vi "MoveMultiDrives.vi"(0 "Start Counter":dbl[](array[numeric]), 1 "Matched Configurations In":T2[](array[typedef]) {"Static Drive Configuration"."Indexer Mode  (FSA)" items=["Incremental", "Absolute"]; "Static Drive Configuration"."Buffer at Stop (SSH)" items=["Clear buffer", "Save and Continue"]; "Static Drive Configuration"."Buffer at Limit (SSG)" items=["Clear buffer", "Save and Continue"]; "Static Drive Configuration"."RS232 Echo Control (SSA)" items=["Echo ON", "Echo OFF"]; "Static Drive Configuration"."Reference edge of Home (OSH)" items=["CW", "CCW"]; "Static Drive Configuration"."Encoder Z for Home (OSD)" items=["Don't use", "Enable"]; "Static Drive Configuration"."Home Switch Sense (OSC)" items=["Normally Open", "Normally Closed"]; "Static Drive Configuration"."Home Position (OSB)" items=["Anywhere in Switch", "Edge of Switch"]; "Static Drive Configuration"."Limit Switch Sense (OSA)" items=["Normally Closed", "Normally Open"]; "Static Drive Configuration"."Limit Disable (LD)" items=["Both Enabled", "CW Disabled", "CCW Disabled", "Both Disabled"]; "Static Drive Configuration"."Stall Detect (FSH)" items=["Disable", "Enable"]; "Static Drive Configuration"."OP2 in Deadband (FSG)" items=["Don't Use", "ACTIVATE"]; "Static Drive Configuration"."Stop on Trigger 3 (FSF)" items=["Ignore", "STOP!"]; "Static Drive Configuration"."Activate OP1 on stall (FSE)" items=["Do not Activate", "ACTIVATE!"]; "Static Drive Configuration"."Stop on Stall (FSD)" items=["Continue", "STOP"]; "Static Drive Configuration"."Position Maintenance (FSC)" items=["Disabled", "Enabled"]; "Static Drive Configuration"."Step Mode  (FSB)" items=["Motor", "Encoder"]; "Static Drive Configuration"."Encoder Resolution (ER)" min=1 max=50000; "Static Drive Configuration"."Dead Band Window (DW)" min=0 max=999999999; "Static Drive Configuration"."Dead Band (DB)" min=0 max=999999999; "Static Drive Configuration"."Correction Gain % (CG)" items=["n/a", "12.5", "25", "37.5", "50", "62.5", "75", "87.5", "100"]; "Channel Properties"."Current Pos" format="%.2f"; "Channel Properties"."Backlash/Eng units" format="%.2f"; "Channel Properties"."Pulses/rev" format="%.2f"; "Channel Properties"."Pos Tolerance" format="%.2f"; "Channel Properties"."Pulses/unit" format="%.2f"; "Channel Properties"."Acc. Min" format="%.2f"; "Channel Properties"."Acc. Max" format="%.2f"; "Channel Properties"."Vel. Min" format="%.2f"; "Channel Properties"."Vel. Max" format="%.2f"; "Channel Properties"."Acc. Default" format="%.2f"; "Channel Properties"."Vel. Default" format="%.2f"}, 2 "GoTo Array (pulse position some channels)":T5[](array[typedef]) {"Acceleration" format="%.2f"; "Velocity" format="%.2f"; "Go To Position" step=100000.0}, 3 "Final move":bool, 4 "Predicted Move Time":dbl format="%.2f") -> (5 "Error string":string, 6 "Stop Pressed?":bool, 7 "Matched Configurations Out":T2[](array[typedef]) {"Static Drive Configuration"."Indexer Mode  (FSA)" items=["Incremental", "Absolute"]; "Static Drive Configuration"."Buffer at Stop (SSH)" items=["Clear buffer", "Save and Continue"]; "Static Drive Configuration"."Buffer at Limit (SSG)" items=["Clear buffer", "Save and Continue"]; "Static Drive Configuration"."RS232 Echo Control (SSA)" items=["Echo ON", "Echo OFF"]; "Static Drive Configuration"."Reference edge of Home (OSH)" items=["CW", "CCW"]; "Static Drive Configuration"."Encoder Z for Home (OSD)" items=["Don't use", "Enable"]; "Static Drive Configuration"."Home Switch Sense (OSC)" items=["Normally Open", "Normally Closed"]; "Static Drive Configuration"."Home Position (OSB)" items=["Anywhere in Switch", "Edge of Switch"]; "Static Drive Configuration"."Limit Switch Sense (OSA)" items=["Normally Closed", "Normally Open"]; "Static Drive Configuration"."Limit Disable (LD)" items=["Both Enabled", "CW Disabled", "CCW Disabled", "Both Disabled"]; "Static Drive Configuration"."Stall Detect (FSH)" items=["Disable", "Enable"]; "Static Drive Configuration"."OP2 in Deadband (FSG)" items=["Don't Use", "ACTIVATE"]; "Static Drive Configuration"."Stop on Trigger 3 (FSF)" items=["Ignore", "STOP!"]; "Static Drive Configuration"."Activate OP1 on stall (FSE)" items=["Do not Activate", "ACTIVATE!"]; "Static Drive Configuration"."Stop on Stall (FSD)" items=["Continue", "STOP"]; "Static Drive Configuration"."Position Maintenance (FSC)" items=["Disabled", "Enabled"]; "Static Drive Configuration"."Step Mode  (FSB)" items=["Motor", "Encoder"]; "Static Drive Configuration"."Encoder Resolution (ER)" min=1 max=50000; "Static Drive Configuration"."Dead Band Window (DW)" min=0 max=999999999; "Static Drive Configuration"."Dead Band (DB)" min=0 max=999999999; "Static Drive Configuration"."Correction Gain % (CG)" items=["n/a", "12.5", "25", "37.5", "50", "62.5", "75", "87.5", "100"]; "Channel Properties"."Current Pos" format="%.2f"; "Channel Properties"."Backlash/Eng units" format="%.2f"; "Channel Properties"."Pulses/rev" format="%.2f"; "Channel Properties"."Pos Tolerance" format="%.2f"; "Channel Properties"."Pulses/unit" format="%.2f"; "Channel Properties"."Acc. Min" format="%.2f"; "Channel Properties"."Acc. Max" format="%.2f"; "Channel Properties"."Vel. Min" format="%.2f"; "Channel Properties"."Vel. Max" format="%.2f"; "Channel Properties"."Acc. Default" format="%.2f"; "Channel Properties"."Vel. Default" format="%.2f"})   [LabVIEW 2010]
uses:
  ~subVIs/DriveClusterLower.ctl
  ~subVIs/AxisConfigCluster.ctl
  ~subVIs/DriveProperties.ctl
  ~subVIs/DriveStaticConfig.ctl
  ~subVIs/DriveStatus.ctl
  ~subVIs/GenericDriveCommand.ctl
  ~subVIs/DriveConfigGlobal.vi
panel:
  out "Server copy Location":path
  out "Log File":path
  out "Move Terminated on Timeout":bool
  in  "Axis info cluster":T1
  out "Start Time":dbl format="%.2f"
  out "Running":bool
  out "Bar2":dbl(slide)=2.0 scale=0.0..-50.0
  out "Bar1":dbl(slide)=2.0 scale=34109.0..-5753.438776987422
  out "Bar0":dbl(slide)=2.0 scale=204595.2..204800.0
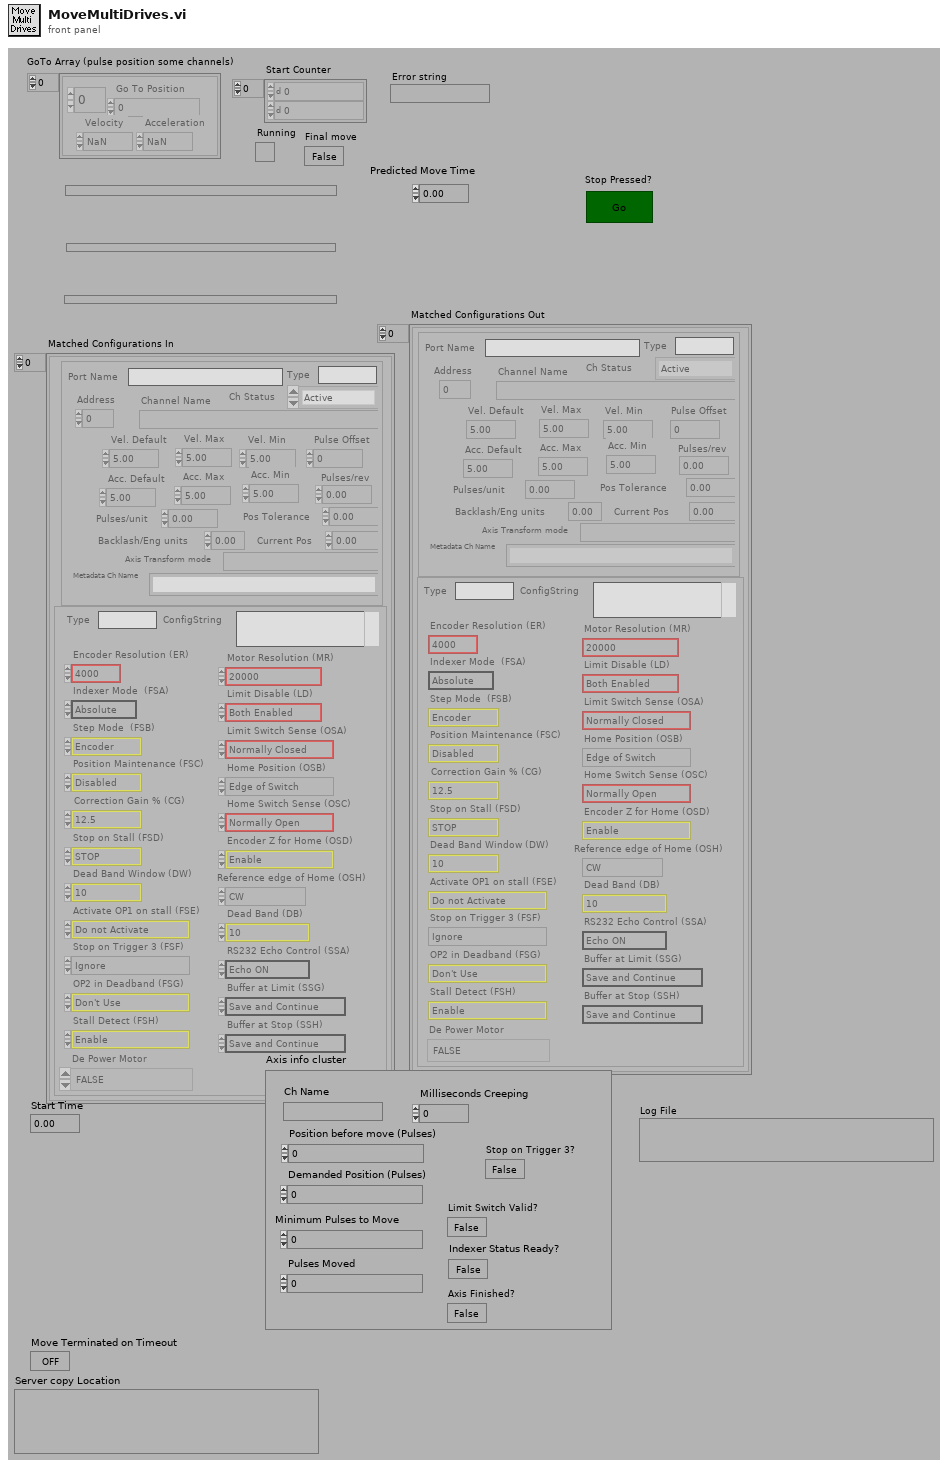
[diagram p1: front panel]
types:
  T1 = typedef "DriveStatus.ctl" = cluster{"Ch Name":string, "Position before move (Pulses)":dbl, "Demanded Position (Pulses)":dbl, "Minimum Pulses to Move":dbl, "Pulses Moved":dbl, "Indexer Status Ready?":bool, "Axis Finished?":bool, "Limit Switch Valid?":bool, "Milliseconds Creeping":u32, "Stop on Trigger 3?":bool}
  T2 = typedef "AxisConfigCluster.ctl" = cluster{"Channel Properties":T3, "Static Drive Configuration":T4}
  T3 = typedef "DriveProperties.ctl" = cluster{"Channel Name":string, "Vel. Default":dbl, "Acc. Default":dbl, "Vel. Max":dbl, "Vel. Min":dbl, "Acc. Max":dbl, "Acc. Min":dbl, "Pulses/unit":dbl, "Address":u8, "Pulse Offset":i32, "Pos Tolerance":dbl, "Pulses/rev":dbl, "Backlash/Eng units":dbl, "Current Pos":dbl, "Ch Status":enum16{"Active", "Offline", "Simulate"}, "Port Name":string, "Axis Transform mode":string, "Metadata Ch Name":string, "Type":string}
  T4 = typedef "DriveStaticConfig.ctl" = cluster{"Correction Gain % (CG)":u16, "Dead Band (DB)":i32, "Dead Band Window (DW)":i32, "Encoder Resolution (ER)":i32, "Step Mode  (FSB)":u16, "Position Maintenance (FSC)":u16, "Stop on Stall (FSD)":u16, "Activate OP1 on stall (FSE)":u16, "Stop on Trigger 3 (FSF)":u16, "OP2 in Deadband (FSG)":u16, "Stall Detect (FSH)":u16, "Limit Disable (LD)":u16, "Motor Resolution (MR)":enum16{"200", "400", "1000", "2000", "4000", "5000", "10000", "12800", "18000", "20000", "21600", "25000", "25400", "25600", "36000", "50000", "278528", "425984", "507904", "614400", "655360", "819200", "1024000"}, "Limit Switch Sense (OSA)":u16, "Home Position (OSB)":u16, "Home Switch Sense (OSC)":u16, "Encoder Z for Home (OSD)":u16, "Reference edge of Home (OSH)":u16, "RS232 Echo Control (SSA)":u16, "Buffer at Limit (SSG)":u16, "Buffer at Stop (SSH)":u16, "Indexer Mode  (FSA)":u16, "Type":string, "ConfigString":string, "De Power Motor":enum16{"TRUE", "FALSE"}}
  T5 = typedef "DriveClusterLower.ctl" = cluster{"Go To Position":dbl, "Velocity":dbl, "Acceleration":dbl, "Address":u8}
  T6 = typedef "GenericDriveCommand.ctl" = string
  T7 = cluster{"GenericDriveCommand":T6, "Go To Position":dbl}
  T8 = cluster{"GenericDriveCommand":T6, "Velocity":dbl}
  T9 = cluster{"GenericDriveCommand":T6, "Acceleration":dbl}
  T10 = cluster{"GenericDriveCommand":T6, "Acceleration":dbl}[]
  T11 = enum16{"A-    Acceleration (rps)", "B-    Buffer Status", "C-    Continue", "CG-  Correction Gain", "CR-  Cariage Return", "D-    Distance (pulses)", "DB-  Dead Band (encoder steps)", "DW- Deadband Window (encoder steps)", "E-    Enable Communications", "ER-  Encoder Resolution (steps/rev)", "F-    Disable Communications", "FS-  Encoder Functions Report", "FSA- Incremental/Absolute (0/1)", "FSB- Motor/Encoder Step Mode (0/1)", "FSC- Enable/Disable Position Maint. (1/0)", "FSD- Stop/Continue on Stall (1/0)", "FSE- Activate o/p1 on Stall (1/0)", "FSF- Stop Motion on Trig3 (1/0)", "FSG- Activate o/p2 in Deadband (1/0)", "FSH- Enable Stall Detect (1/0)", "G- Go", "GH- Go Home and Zero (+/-V)", "^H- Delete ", "H- Direction Reverse/CCW/CW (0,1,2)", "IS- Input Status", "K- Kill", "L- Loop (n)", "LD- Limit DISABLE (0-none,1-CW,2-CCW,3-Both)", "LF- Line Feed", "MC- Mode Continuous", "MN- Mode Normal", "MPA- Motor Postion Absolute", "MPI- Motor Position Incremental", "MR- Motor Resolution (Drive Steps/rev)", "N- End of Loop", "O- Output (00,01,10,11)", "OS- Report Homing Setup", "OSA- NO/NC Limits (1/0)", "OSB- Back Up to Home/Edge? (0/1)", "OSC- NO/NC Home Switch (1/0)", "OSD- Enable Encoder Z for Home (0/1)", "OSH- Reference Edge for Home CW/CCW (0/1)", "PR- Report ABSOLUTE Position", "PS- Pause until Continue", "PX- Report Absolute ENCODER Position", "PZ- Zero Absolute Counter", "\"- Quote (17 ASCII +Space)", "Q- Enter/Exit Velocity Profiling (1/0)", "R- Request Indexer Status", "RA- Report Limit Switch Status", "RB- Report Loop, Pause, Shutdown, Trigger Status", "RC- Report Closed Loop Status", "RM- Velocity Streaming Rate Multiplier (000-FFF)", "RV- Report Revision Level", "S- Controlled Stop", "SN- Debounce (1-1000ms)", "SS- Report Software Switch Status", "SSA- Disable RS232 Echo (1/0)", "SSG- Clear/Save Command Buffer on Limit (0/1)", "SSH- Clear/Save Command Buffer on Stop (0/1)", "ST- Shutdown (1/0)", "SV- Servoing Setting (0,1,2,3)", "T- Time Delay (0.01-99999.99)", "TR- Wait for Trigger High/Low/Ignore (1/0/X)", "TS- Report Trigger Status", "U- Pause after Move Until Continue", "V- Velocity (0.01-50.00 revs/sec)", "W1- Report Relative Position <Signed Binary>", "W3- Report Relative Position <Hexadecimal>", "Y- Abort Loop at N", "Z-    Reset to Defaults", "#-    Disable/Set Soft Addresses (0/1-255)"}
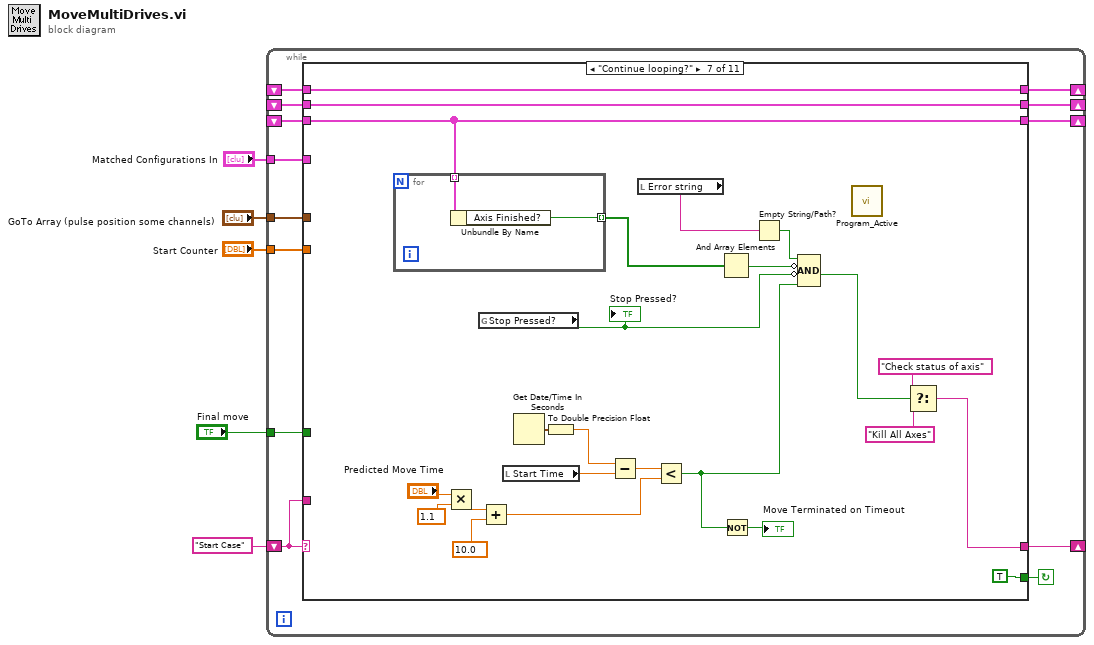
[diagram p0: block diagram]
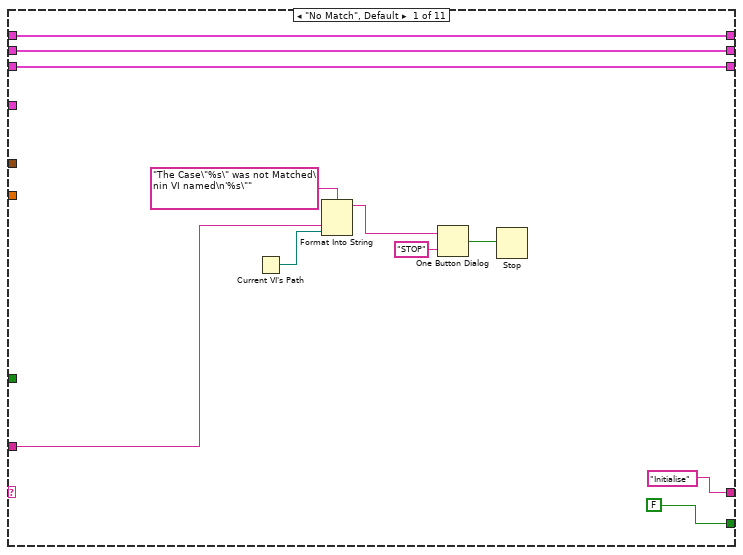
[diagram p2: hidden frame]
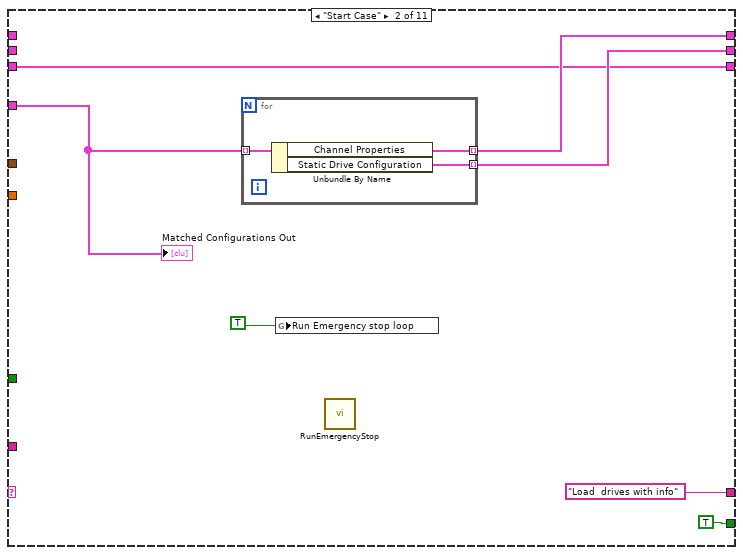
[diagram p3: hidden frame]
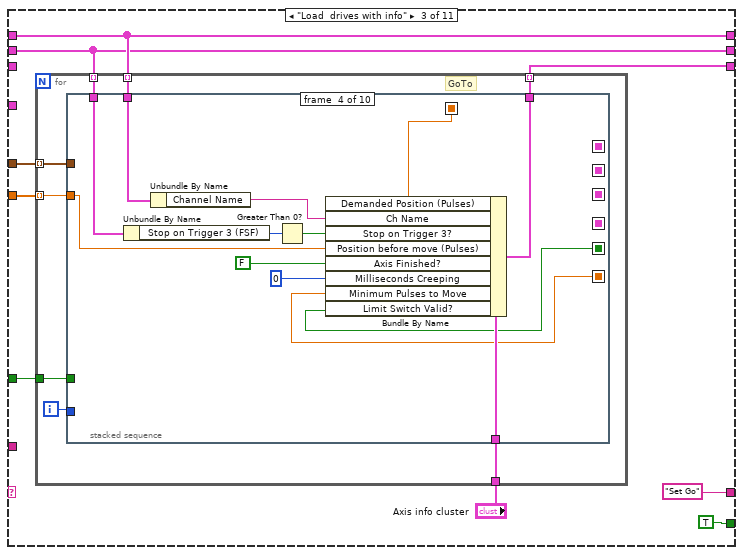
[diagram p4: hidden frame]
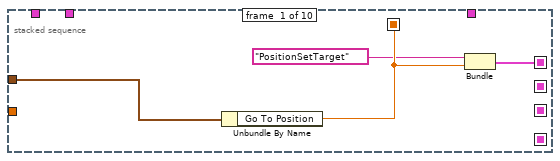
[diagram p5: hidden frame]
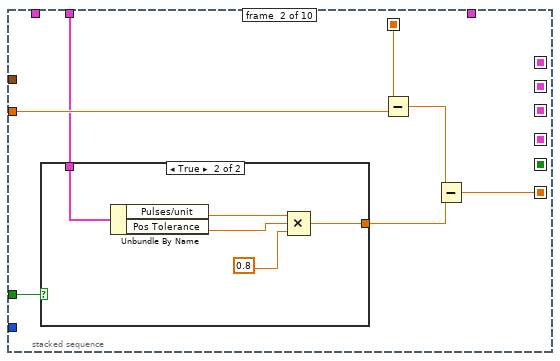
[diagram p6: hidden frame]
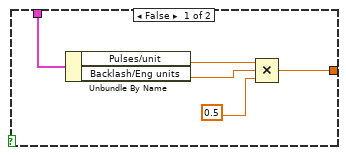
[diagram p7: hidden frame]
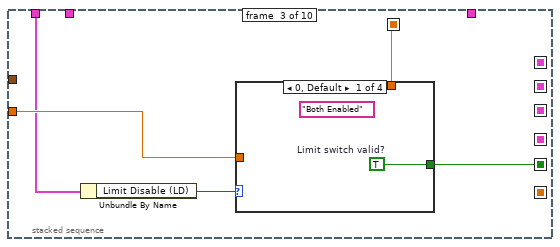
[diagram p8: hidden frame]
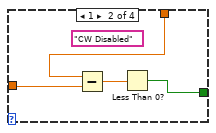
[diagram p9: hidden frame]
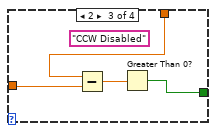
[diagram p10: hidden frame]
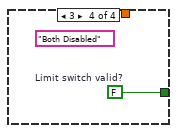
[diagram p11: hidden frame]
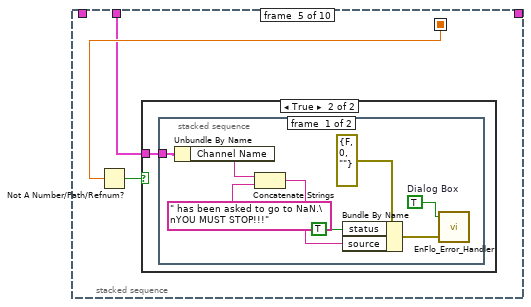
[diagram p12: hidden frame]
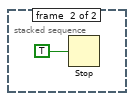
[diagram p14: hidden frame]
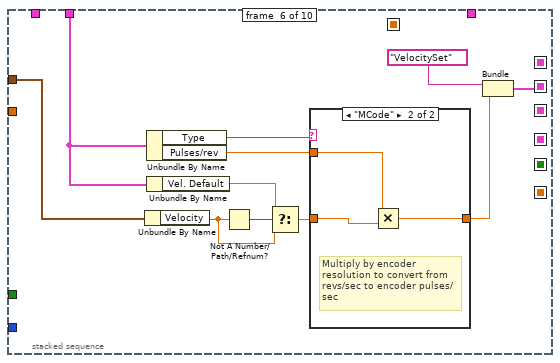
[diagram p15: hidden frame]
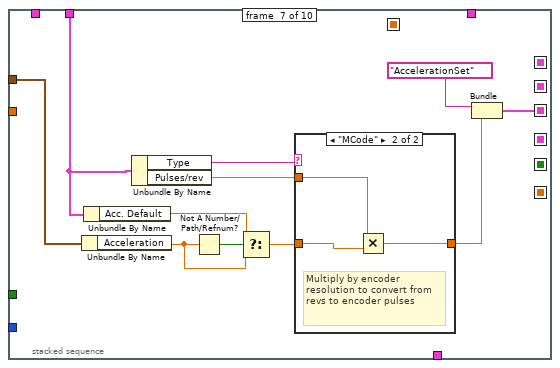
[diagram p17: hidden frame]
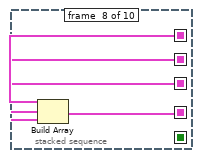
[diagram p19: hidden frame]
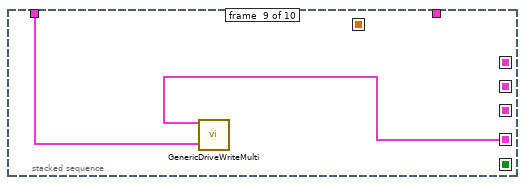
[diagram p20: hidden frame]
diagram:
  n1 = while {
    shift-left: _ -> [w7]
    shift-right: [w6] -> _
    tunnel: "Final move" -> [w8]
    tunnel: "Start Counter" -> [w9]
    tunnel: "GoTo Array (pulse position some channels)" -> [w10]
    tunnel: "Matched Configurations In" -> [w15]
    shift-left: _ -> [w11]
    shift-right: [w13] -> _
    shift-left: _ -> [w12]
    shift-right: [w14] -> _
    shift-left: "Start Case" -> [w16]
    shift-right: [w17] -> _
    stop <- w18 continue-if-true
    n2 = case shown="\"Continue looping?\"" w16 {
      tunnel: [FALSE TRUE TRUE TRUE TRUE TRUE TRUE TRUE TRUE TRUE FALSE] -> w18
      tunnel: ["Initialise" "Load  drives with info" "Set Go" "Record Time" "Check status of axis" "Continue looping?" w224 "Does Log file Exist" w266 "Write to Log file" "End"] -> w17
      tunnel: w16 -> [w24 _ _ _ _ _ _ _ _ _ _]
      tunnel: w15 -> [_ w30 _ w172 _ _ _ _ _ _ _]
      tunnel: [w21 w33 w45 w176 w187 w194 w243 w255 w271 w292 w319] -> w14
      tunnel: [w20 w32 w42 w175 w186 w195 w242 w254 w270 w291 w318] -> w13
      tunnel: w12 -> [w21 _ w45 w176 w187 w194 w243 w255 w271 w292 w319]
      tunnel: w11 -> [w20 _ w42 w175 w186 w195 w242 w254 w270 w291 w318]
      tunnel: w10 -> [_ _ w46 _ _ _ _ _ _ _ _]
      tunnel: w9 -> [_ _ w44 _ _ _ _ _ _ _ _]
      tunnel: w8 -> [_ _ w43 _ _ _ _ _ _ _ _]
      tunnel: [w19 w31 w40 w173 w184 w190 w229 w253 w269 w290 w316] -> w6
      tunnel: w7 -> [w19 w31 _ w173 w184 w191 w229 w253 w269 w290 w316]
      frame "No Match", Default {
        n3 = Current VI's Path() -> (path=w23:path)
        n4 = Format Into String(format string="The Case\"%s\" was not Matched\nin VI named\n'%s\"" ("Format String"), w24, w23) -> (resulting string=w27:string)  [unwired: 2 in, 1 out]
        n5 = One Button Dialog(message=w27, button name ("OK")="STOP") -> (true=w25:bool)
        n6 = Stop(stop? (T)=w25) -> ()
      }
      frame "Start Case" {
        n7 = for {
          tunnel: w30 -> [w39] mode=indexing
          tunnel: [w38] -> w33 mode=indexing
          tunnel: [w37] -> w32 mode=indexing
          n8 = Unbundle By Name(w39) -> ("Channel Properties"=w38:T3, "Static Drive Configuration"=w37:T4)
        }
        n9 = global write "DriveConfigGlobal.vi" "Run Emergency stop loop"(TRUE) -> ()
        n10 = call "RunEmergencyStop.vi"() -> ()  [unwired: 1 in, 7 out]
        "Matched Configurations Out" <- w30
      }
      frame "Load  drives with info" {
        n11 = for {
          tunnel: w46 -> [w55] mode=indexing
          tunnel: w45 -> [w54] mode=indexing
          tunnel: w44 -> [w53] mode=indexing
          tunnel: w43 -> [w52]
          tunnel: w42 -> [w51] mode=indexing
          tunnel: "Axis info cluster" -> [w50]
          tunnel: [w49] -> w40 mode=indexing
          i -> [w56]
          # "GoTo"
          n12 = stacked-sequence {
            seq-local: [w59 _ _ _ _ _ _ _ _ _] -> [_ w67 w81 w96 w108 _ _ _ _ w158]
            seq-local: [w58 _ _ _ _ _ _ _ _ _] -> [_ _ _ _ _ _ _ w152 _ _]
            seq-local: [_ _ _ _ _ w125 _ _ _ _] -> [_ _ _ _ _ _ _ w151 _ _]
            seq-local: [_ _ _ _ _ _ w140 _ _ _] -> [_ _ _ _ _ _ _ w150 _ _]
            seq-local: [_ _ _ _ _ _ _ w149 _ _] -> [_ _ _ _ _ _ _ _ w154 _]
            seq-local: [_ w62 _ _ _ _ _ _ _ _] -> [_ _ _ w103 _ _ _ _ _ _]
            seq-local: [_ _ w78 _ _ _ _ _ _ _] -> [_ _ _ w101 _ _ _ _ _ _]
            tunnel: w55 -> [w60 _ _ _ _ w129 w144 _ _ _]
            tunnel: w56 -> [_ _ _ _ _ _ _ _ _ w155]
            tunnel: w52 -> [_ w65 _ _ _ _ _ _ _ _]
            tunnel: w54 -> [_ w63 _ w105 w106 w123 w138 _ w153 _]
            tunnel: w53 -> [_ w64 w80 w98 _ _ _ _ _ w156]
            tunnel: w51 -> [_ _ w79 w100 _ _ _ _ _ _]
            tunnel: w50 -> [_ _ _ w104 _ _ _ _ _ _]
            tunnel: [_ _ _ w102 _ _ _ _ _ _] -> w49
            frame #0 {
              n13 = Unbundle By Name(w60) -> ("Go To Position"=w59:dbl)
              n14 = Bundle("GenericDriveCommand"=T6 "PositionSetTarget", "Go To Position"=w59) -> (w58:T7)  [unwired: 1 out]
            }
            frame #1 {
              n15 = case shown="True" w65 {
                tunnel: w63 -> [w72 w77]
                tunnel: [w68 w73] -> w66
                frame False {
                  n16 = Unbundle By Name(w72) -> ("Pulses/unit"=w71:dbl, "Backlash/Eng units"=w70:dbl)
                  n17 = Compound Arithmetic op=MULTIPLY(w71, w70, 0.5) -> (w68:dbl)
                }
                frame True {
                  n18 = Unbundle By Name(w77) -> ("Pulses/unit"=w76:dbl, "Pos Tolerance"=w75:dbl)
                  n19 = Compound Arithmetic op=MULTIPLY(w76, w75, 0.8) -> (w73:dbl)
                }
              }
              n20 = Subtract(x=w67, y=w64) -> (x-y=w61:dbl)
              n21 = Subtract(x=w61, y=w66) -> (x-y=w62:dbl)
            }
            frame #2 {
              n22 = Unbundle By Name(w79) -> ("Limit Disable (LD)"=w82:u16)
              n23 = case shown="0, Default" w82 {
                tunnel: [w83 w84 w88 w92] -> w78
                tunnel: w80 -> [_ w86 w90 _]
                tunnel: w81 -> [_ w87 w91 _]
                frame 0, Default {
                  w83 = TRUE  # Limit switch valid?
                  (unwired) "Both Enabled"
                }
                frame 1 {
                  (unwired) "CW Disabled"
                  n24 = Subtract(x=w87, y=w86) -> (x-y=w85:dbl)
                  n25 = Less Than 0?(x=w85) -> (x < 0?=w84:bool)
                }
                frame 2 {
                  (unwired) "CCW Disabled"
                  n26 = Subtract(x=w91, y=w90) -> (x-y=w89:dbl)
                  n27 = Greater Than 0?(x=w89) -> (x > 0?=w88:bool)
                }
                frame 3 {
                  (unwired) "Both Disabled"
                  w92 = FALSE  # Limit switch valid?
                }
              }
            }
            frame #3 {
              n28 = Unbundle By Name(w100) -> ("Stop on Trigger 3 (FSF)"=w99:u16)
              n29 = Unbundle By Name(w105) -> ("Channel Name"=w97:string)
              n30 = Greater Than 0?(x=w99) -> (x > 0?=w95:bool)
              n31 = Bundle By Name(cluster=w104, "Demanded Position (Pulses)"=w96, "Ch Name"=w97, "Stop on Trigger 3?"=w95, "Position before move (Pulses)"=w98, "Axis Finished?"=FALSE ("Bundle Element"), "Milliseconds Creeping"=u32 0 ("Bundle Element"), "Minimum Pulses to Move"=w103, "Limit Switch Valid?"=w101) -> (w102:T1)
            }
            frame #4 {
              n32 = Not A Number/Path/Refnum?(number/path/refnum=w108) -> (NaN/Path/Refnum?=w107:bool)
              n33 = case shown="True" w107 {
                tunnel: w106 -> [_ w109]
                frame False {
                }
                frame True {
                  n34 = stacked-sequence {
                    tunnel: w109 -> [w117 _]
                    frame #0 {
                      w110 = TRUE  # Dialog Box
                      n35 = Unbundle By Name(w117) -> ("Channel Name"=w113:string)
                      n36 = Concatenate Strings(w113, " has been asked to go to NaN.\nYOU MUST STOP!!!") -> (w111:string)
                      n37 = Bundle By Name(cluster=errorcluster {"status"=FALSE, "code"=0, "source"=""} ("error in (no error)"), "status"=TRUE ("Bundle Element"), "source"=w111) -> (w115:errorcluster)
                      n38 = call "EnFlo_Error_Handler.vi"("error in (no error)"=w115, "Dialog Box (T)"=w110) -> ()  [unwired: 1 in, 3 out]
                    }
                    frame #1 {
                      n39 = Stop(stop? (T)=TRUE) -> ()
                    }
                  }
                }
              }
            }
            frame #5 {
              n40 = Unbundle By Name(w129) -> ("Velocity"=w126:dbl)
              n41 = Unbundle By Name(w123) -> ("Type"=w122:string, "Pulses/rev"=w120:dbl)
              n42 = Unbundle By Name(w123) -> ("Vel. Default"=w127:dbl)
              n43 = Not A Number/Path/Refnum?(number/path/refnum=w126) -> (NaN/Path/Refnum?=w128:bool)
              n44 = Select(t=w127, s=w128, f=w126) -> (s? t:f=w121:dbl)
              n45 = case shown="\"MCode\"" w122 {
                tunnel: w121 -> [w130 w133]
                tunnel: w120 -> [_ w132]
                tunnel: [w130 w131] -> w119
                frame "ParkerX", Default {
                }
                frame "MCode" {
                  # "Multiply by encoder resolution to convert from revs/sec to encoder pulses/sec"
                  n46 = Multiply(x=w132, y=w133) -> (x*y=w131:dbl)
                }
              }
              n47 = Bundle("GenericDriveCommand"=T6 "VelocitySet", "Velocity"=w119) -> (w125:T8)  [unwired: 1 out]
            }
            frame #6 {
              n48 = Unbundle By Name(w144) -> ("Acceleration"=w141:dbl)
              n49 = Unbundle By Name(w138) -> ("Acc. Default"=w142:dbl)
              n50 = Unbundle By Name(w138) -> ("Type"=w137:string, "Pulses/rev"=w136:dbl)
              n51 = Not A Number/Path/Refnum?(number/path/refnum=w141) -> (NaN/Path/Refnum?=w143:bool)
              n52 = Select(t=w142, s=w143, f=w141) -> (s? t:f=w135:dbl)
              n53 = case shown="\"MCode\"" w137 {
                tunnel: w135 -> [w145 w148]
                tunnel: w136 -> [_ w147]
                tunnel: [w145 w146] -> w134
                frame "ParkerX", Default {
                }
                frame "MCode" {
                  # "Multiply by encoder resolution to convert from revs to encoder pulses"
                  n54 = Multiply(x=w147, y=w148) -> (x*y=w146:dbl)
                }
              }
              n55 = Bundle("GenericDriveCommand"=T6 "AccelerationSet", "Acceleration"=w134) -> (w140:T9)  [unwired: 1 out]
            }
            frame #7 {
              n56 = Build Array(w152, w151, w150) -> (w149:T10)
            }
            frame #8 {
              n57 = call "GenericDriveWriteMulti.vi"("Channel Description"=w153, "Array Constant"=w154) -> ()  [unwired: 1 out]
            }
            frame #9 {
              n58 = Max & Min(x=w158, y=w156) -> (max(x,y)=w160:dbl, min(x,y)=w159:dbl)
              n59 = Less?(x=w158, y=w156) -> (x < y?=w157:bool)
              n60 = case shown="0, Default" w155 {
                tunnel: w160 -> [w163 w166 w169]
                tunnel: w159 -> [w162 w165 w168]
                tunnel: w157 -> [w161 w164 w167]
                frame 0, Default {
                  n61 = property on="Bar0" class="Slide (strict)"("Scale.Range:Maximum"=w163, "Scale.Range:Minimum"=w162, "Scale.Flipped"=w161) -> ()  [unwired: 2 in, 2 out]
                }
                frame 1 {
                  n62 = property on="Bar1" class="Slide (strict)"("Scale.Range:Maximum"=w166, "Scale.Range:Minimum"=w165, "Scale.Flipped"=w164) -> ()  [unwired: 2 in, 2 out]
                }
                frame 2 {
                  n63 = property on="Bar2" class="Slide (strict)"("Scale.Range:Maximum"=w169, "Scale.Range:Minimum"=w168, "Scale.Flipped"=w167) -> ()  [unwired: 2 in, 2 out]
                }
              }
            }
          }
        }
      }
      frame "Set Go" {
        n64 = call "GetActivePortNames.vi"("Matched Configurations In"=w172) -> ("Port Name Array"=w171:string[], "Drive Type Array"=w170:string[])
        n65 = for {
          tunnel: w171 -> [w182] mode=indexing
          tunnel: "Global" -> [w181]
          tunnel: w170 -> [w180] mode=indexing
          n66 = call "GenericDriveIO.vi"("GenericDriveCommand"=T6 "GoNow", "Channel Name"=w181, "Type"=w180, "Port Name"=w182) -> ()  [unwired: 2 in, 6 out]
        }
      }
      frame "Record Time" {
        n67 = Get Date/Time In Seconds() -> (seconds since 1Jan1904=w183:timestamp)
        n68 = To Double Precision Float(number=w183) -> (double precision float=→"Start Time":dbl)
      }
      frame "Check status of axis" {
        (unwired) "Global"
        n69 = for {
          shift-right: [w202] -> w192
          shift-left: "" -> [w204]
          tunnel: w194 -> [w203] mode=indexing
          tunnel: w191 -> [w199] mode=indexing
          tunnel: [w198] -> w190 mode=indexing
          i -> [w205]
          n70 = Unbundle By Name(w199) -> ("Axis Finished?"=w200:bool, "Position before move (Pulses)"=w201:dbl)
          n71 = case shown="False" w200 {
            tunnel: w205 -> [w215 _]
            tunnel: w204 -> [w214 w220]
            tunnel: w203 -> [w212 _]
            tunnel: [w211 w220] -> w202
            tunnel: w201 -> [w210 _]
            tunnel: w199 -> [w209 w219]
            tunnel: [w206 w219] -> w198
            frame False {
              n72 = call "CheckDriveStatus.vi"("Channel Properties"=w212, "Axis info cluster"=w209) -> ("Error string"=w213:string, "Axis info cluster Out"=w206:T1)
              n73 = Unbundle By Name(w206) -> ("Pulses Moved"=w208:dbl)
              n74 = Add(x=w210, y=w208) -> (x+y=w207:dbl)
              n75 = case shown="2" w215 {
                tunnel: w207 -> [w216 w217 w218]
                frame 0, Default {
                  "Bar0" <- w216
                }
                frame 1 {
                  "Bar1" <- w217
                }
                frame 2 {
                  "Bar2" <- w218
                }
              }
              n76 = Concatenate Strings(w214, w213) -> (w211:string)
            }
            frame True {
            }
          }
        }
        "Error string" <- w192
      }
      frame "Continue looping?" {
        n77 = for {
          tunnel: w229 -> [w246] mode=indexing
          tunnel: [w245] -> w228 mode=indexing
          n78 = Unbundle By Name(w246) -> ("Axis Finished?"=w245:bool)
        }
        n79 = Multiply(x="Predicted Move Time", y=1.1) -> (x*y=w235:dbl)
        n80 = global read "DriveConfigGlobal.vi" "Stop Pressed?"() -> (w238:bool)
        "Stop Pressed?" <- w238
        n81 = Add(x=w235, y=10.0) -> (x+y=w231:dbl)
        n82 = local read "Start Time"() -> (w230:dbl)
        n83 = Get Date/Time In Seconds() -> (seconds since 1Jan1904=w221:timestamp)
        n84 = To Double Precision Float(number=w221) -> (double precision float=w236:dbl)
        n85 = Subtract(x=w236, y=w230) -> (x-y=w237:dbl)
        n86 = local read "Error string"() -> (w239:string)
        n87 = Less?(x=w237, y=w231) -> (x < y?=w223:bool)
        n88 = And Array Elements(Boolean array=w228) -> (logical AND=w241:bool)
        n89 = Not(x=w223) -> (.not. x?=→"Move Terminated on Timeout":bool)
        n90 = Empty String/Path?(string/path=w239) -> (empty?=w240:bool)
        n91 = Compound Arithmetic op=AND(w240, invert w241, invert w238, w223) -> (w227:bool)
        n92 = call "Program_Active.vi"() -> ()  [unwired: 1 in]
        n93 = Select(t="Check status of axis", s=w227, f="Kill All Axes") -> (s? t:f=w224:string)
      }
      frame "Kill All Axes" {
        # "Kill All Axis in case they are creeping"
        n94 = global read "DriveConfigGlobal.vi" "Configurations"() -> (w252:T2[])
        n95 = call "GetActivePortNames.vi"("Matched Configurations In"=w252) -> ("Port Name Array"=w249:string[], "Drive Type Array"=w247:string[])
        n96 = for {
          tunnel: w249 -> [w260] mode=indexing
          tunnel: "Global" -> [w259]
          tunnel: w247 -> [w258] mode=indexing
          (unwired) T11."K- Kill" ("COMMAND")
          n97 = call "GenericDriveIO.vi"("GenericDriveCommand"=T6 "StopEmergency", "Channel Name"=w259, "Type"=w258, "Port Name"=w260) -> ()  [unwired: 2 in, 6 out]
        }
        "Running" <- FALSE
      }
      frame "Does Log file Exist" {
        n98 = call "Create_Error_log_folders.vi"("Per Day Log File?"=TRUE, "Log Filename"="Traverse_Low" ("Input Element")) -> ("exists?"=w263:bool, "Server copy Location"=→"Server copy Location":path, "Local Log File"=→"Log File":path)  [unwired: 1 in]
        n99 = Select(t="Write to Log file", s=w263, f="Create Log file") -> (s? t:f=w266:string)
      }
      frame "Create Log file" {
        n100 = Build Array("Date::", "Time::", "Seconds:Since:1st Jan 1904", "Move:Duration:Seconds", "Move:Terminated:On Timeout") -> (w281:string[])
        n101 = for {
          N: 3 -> [_]
          shift-right: [w294] -> w280
          shift-left: w281 -> [w295]
          i -> [w300]
          n102 = Increment(x=w300) -> (x+1=w299:i32)
          n103 = Number To Decimal String(number=w299) -> (decimal integer string=w298:string)  [unwired: 1 out]
          n104 = Build Array("Axis:Ch Name:", "Position Before:Move (Pulses):", "Demanded:Position (Pulses):", "Minimum Pulses:to Move:", "Pulses:Moved:", "Indexer:Status Ready:", "Axis:Finished?", "Limit:Switch Valid?") -> (w297:string[])
          n105 = for {
            tunnel: w298 -> [w311]
            tunnel: w297 -> [w310] mode=indexing
            tunnel: [w309] -> w296 mode=indexing
            n106 = Concatenate Strings(w310, w311) -> (w309:string)
          }
          n107 = Build Array (concatenate)(w295, w296) -> (w294:string[])
        }
        n108 = for {
          tunnel: w280 -> [w315] mode=indexing
          tunnel: [w314] -> w284 mode=indexing
          tunnel: [w313] -> w285 mode=indexing
          tunnel: [w312] -> w286 mode=indexing
          n109 = call "Split_Ch_name.vi"("Ch name"=w315) -> ("Top level"=w314:string, "Middle"=w313:string, "Low level"=w312:string)
        }
        n110 = local read "Log File"() -> (w273:path)
        n111 = Build Array(w284, w285, w286) -> (w282:string[][])
        n112 = Array To Spreadsheet String(array=w282, 3:"%s" ("format string")) -> (spreadsheet string=w274:string)  [unwired: 1 out]
        n113 = call "Write_File_Simple.vi"("append to file? (new file:F)"=TRUE, "character string"=w274, "file path"=w273) -> ()  [unwired: 2 out]
      }
      frame "Write to Log file" {
        n114 = stacked-sequence {
          seq-local: [w325 _ _] -> [_ w337 _]
          seq-local: [_ w336 _] -> [_ _ w363]
          tunnel: w316 -> [_ w338 _]
          frame #0 {
            n115 = local read "Move Terminated on Timeout"() -> (w332:bool)
            n116 = Get Date/Time In Seconds() -> (seconds since 1Jan1904=w324:timestamp)
            n117 = local read "Start Time"() -> (w334:dbl)
            n118 = To Double Precision Float(number=w324) -> (double precision float=w323:dbl)
            n119 = Subtract(x=w323, y=w334) -> (x-y=w333:dbl)
            n120 = Get Date/Time String(date format (0)=enum16{"short", "long", "abbreviated"}."abbreviated", seconds (now)=w324) -> (date string=w329:string, time string=w328:string)  [unwired: 1 out]
            n121 = Number To Fractional String(number=w323, precision (6)=i16 3) -> (F-format string=w321:string)  [unwired: 2 out]
            n122 = Number To Decimal String(number=w333) -> (decimal integer string=w327:string)  [unwired: 1 out]
            n123 = Select(t="TRUE", s=w332, f="FALSE") -> (s? t:f=w326:string)
            n124 = Build Array(w329, w328, w321, w327, w326) -> (w325:string[])
          }
          frame #1 {
            n125 = for {
              tunnel: w338 -> [w353] mode=indexing
              shift-right: [w341] -> w336
              shift-left: w337 -> [w342]
              n126 = Unbundle By Name(w353) -> ("Ch Name"=w345:string, "Position before move (Pulses)"=w352:dbl, "Demanded Position (Pulses)"=w351:dbl, "Minimum Pulses to Move"=w339:dbl, "Pulses Moved"=w350:dbl, "Indexer Status Ready?"=w349:bool, "Axis Finished?"=w348:bool, "Limit Switch Valid?"=w340:bool)
              n127 = Build Array(w352, w351, w339, w350) -> (w346:dbl[])
              n128 = Build Array(w349, w348, w340) -> (w347:bool[])
              n129 = Number To Decimal String(number=w346) -> (decimal integer string=w344:string[])  [unwired: 1 out]
              n130 = for {
                tunnel: w347 -> [w355] mode=indexing
                tunnel: [w354] -> w343 mode=indexing
                n131 = Select(t="TRUE", s=w355, f="FALSE") -> (s? t:f=w354:string)
              }
              n132 = Build Array (concatenate)(w342, w345, w344, w343) -> (w341:string[])
            }
          }
          frame #2 {
            n133 = for {
              shift-right: [w367] -> w360
              shift-left: "\r" -> [w368]
              tunnel: w363 -> [w366] mode=indexing
              n134 = Concatenate Strings(w368, w366, "\t") -> (w367:string)
            }
            n135 = local read "Log File"() -> (w361:path)
            n136 = local read "Server copy Location"() -> (w359:path)
            n137 = call "Write_File_Simple.vi"("append to file? (new file:F)"=TRUE, "character string"=w360, "file path"=w361) -> ("file path Out"=w358:path)  [unwired: 1 out]
            n138 = call "Updated_File_Copy.vi"("Target Path"=w359, "Source Path"=w358) -> ()  [unwired: 2 out]
          }
        }
      }
    }
  }
